vi "JSONPath to Excel Named Range.vi"(8 "error in":errorcluster, 11 "JSONPath":string) -> (0 "error out":errorcluster, 3 "Named Range":string)   [LabVIEW 2019, in "Config from Excel Table.lvclass"]
uses:
  Config from Excel Table.lvclass
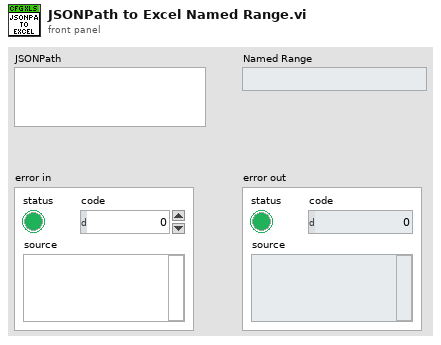
[diagram p1: front panel]
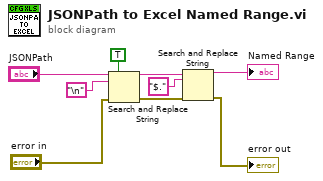
[diagram p0: block diagram]
diagram:
  n1 = Search and Replace String(replace all?=TRUE ("replace all? (F)"), input string="JSONPath", search string="\n", error in="error in") -> (result string=w4:string, error out=w2:errorcluster)  [unwired: 4 in, 2 out]
  n2 = Search and Replace String(input string=w4, search string="$." ("search string/char (-)"), error in=w2) -> (result string=→"Named Range":string, error out=→"error out":errorcluster)  [unwired: 5 in, 2 out]
